vi "Drive Time.vi"(6 "Force? (F)":bool, 7 "Wait for Completion? (F)":bool, 8 "error in":errorcluster, 9 "Y Axis":dbl, 10 "X Axis":dbl, 11 "Time (ms)":u32) -> (0 "error out":errorcluster)   [LabVIEW 2016, in "Drive System.lvlib"]
uses:
  Drive System.lvlib
  Private/DriveCmd.ctl
  Private/DriveCmdList.ctl
  Private/Varient Cmd Types/Drive Time.ctl
panel:
  in  "Timeout ms (-1)":i32=-1
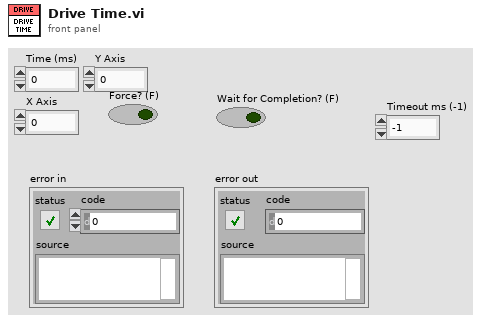
[diagram p1: front panel]
types:
  T1 = typedef "Drive System.lvlib/Drive Time.ctl" = cluster{"X Axis":dbl, "Y Axis":dbl, "Time (ms)":u32}
  T2 = typedef "Drive System.lvlib/DriveCmd.ctl" = cluster{"cmd":T3, "data":variant, "Force? (F)":bool, "Lock":string}
  T3 = typedef "Drive System.lvlib/DriveCmdList.ctl" = enum16{"Idle", "Cleanup", "Drive For Time", "Follow Path", "Drive Tank", "Drive Arcade", "Unlock", "Lock"}
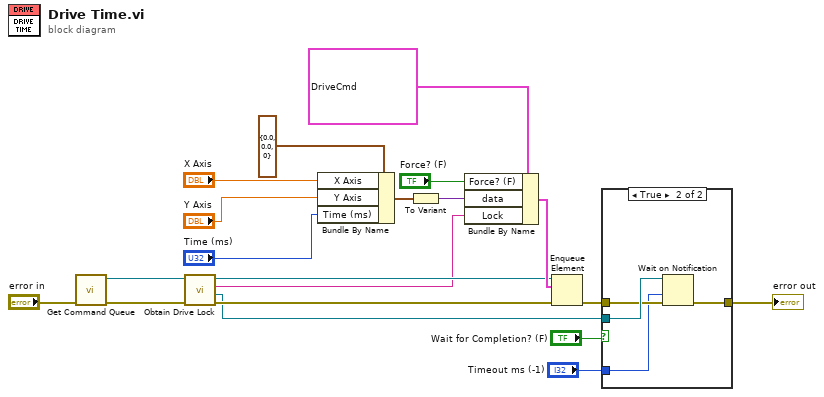
[diagram p0: block diagram]
diagram:
  n1 = call "Get Command Queue.vi"("error in (no error)"="error in") -> ("error out"=w20:errorcluster, "Queue out"=w19:refnum<queue>)  [unwired: 9 in]
  n2 = call "Obtain Drive Lock.vi"("error in"=w20, "Queue in"=w19) -> ("error out"=w12:errorcluster, "notifier out"=w3:refnum<notifier>, "Lock"=w6:string, "queue out"=w11:refnum<queue>)  [unwired: 6 in]
  n3 = Bundle By Name(cluster=T1 {"X Axis"=0.0, "Y Axis"=0.0, "Time (ms)"=0} ("Cluster"), "X Axis"="X Axis", "Y Axis"="Y Axis", "Time (ms)"="Time (ms)") -> (w15:T1)
  n4 = To Variant(anything=w15) -> (Variant=w16:variant)
  n5 = Bundle By Name(cluster=T2 {"cmd"=enum."Drive For Time", "data"=variant, "Force? (F)"=FALSE, "Lock"=""} ("element"), "Force? (F)"="Force? (F)", "data"=w16, "Lock"=w6) -> (w17:T2)
  n6 = Enqueue Element(queue=w11, element=w17, error in (no error)=w12) -> (error out=w4:errorcluster)  [unwired: 1 in, 2 out]
  n7 = case shown="True" "Wait for Completion? (F)" {
    tunnel: w4 -> [w21 w24]
    tunnel: w3 -> [_ w25]
    tunnel: [w21 w23] -> w2
    tunnel: "Timeout ms (-1)" -> [_ w22]
    frame False {
    }
    frame True {
      n8 = Wait on Notification(notifier=w25, timeout in ms (-1)=w22, error in (no error)=w24) -> (error out=w23:errorcluster)  [unwired: 1 in, 3 out]
    }
  }
  "error out" <- w2
